vi "SenddPWMProtocol.vi"(7 "Send":bool, 9 "Initialize":bool, 10 "Tmpl values":T1={"type"="AI", "device"="", "name"="", "data"={"<init"=FALSE, "<duty_cycle"=0.0, "<dio_pin"=0.0}}, 11 "Tmpl values":T1={"type"="AI", "device"="", "name"="", "data"={"<init"=FALSE, "<duty_cycle"=0.0, "<dio_pin"=0.0}}) -> ()   [LabVIEW 2019]
uses:
  dPWM proto.ctl
  dPWM Data proto.ctl
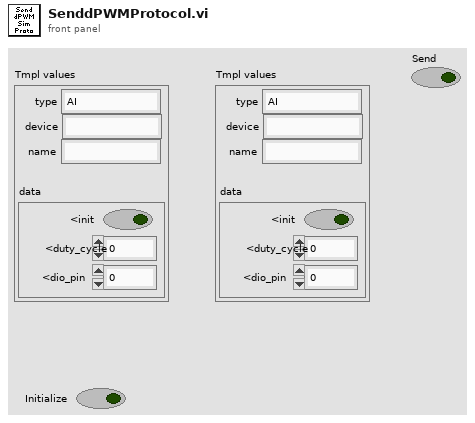
[diagram p1: front panel]
types:
  T1 = typedef "dPWM proto.ctl" = cluster{"type":string, "device":string, "name":string, "data":T2}
  T2 = typedef "dPWM Data proto.ctl" = cluster{"<init":bool, "<duty_cycle":dbl, "<dio_pin":dbl}
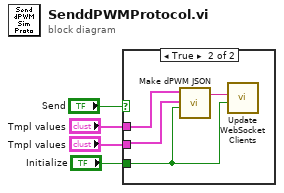
[diagram p0: block diagram]
diagram:
  n1 = case shown="True" "Send" {
    tunnel: "Tmpl values" -> [_ w8]
    tunnel: "Tmpl values" -> [_ w7]
    tunnel: "Initialize" -> [_ w6]
    frame False {
    }
    frame True {
      n2 = call "Make dPWM JSON.vi"("Force"=w6, 10:"Tmpl values"=w7, 11:"Tmpl values"=w8) -> ("delta JSON"=w5:string)  [unwired: 8 in]
      n3 = call "Update WebSocket Clients.vi"("Initialize"=w6, "delta JSON"=w5) -> ()  [unwired: 10 in]
    }
  }
